vi "GUI.vi"() -> ()   [LabVIEW 2024]
uses:
  <vilib>/Python/Open Anaconda Python Session.vi
panel:
  out "转换完成":bool
  in  "开始转换":bool
  out "运行中":bool
  in  "OCR all pages":bool
  in  "Batch_multiplier":i32(slide) scale=0.0..8.0
  in  "Start page":i32
  in  "Max pages":i32
  in  "PDF directory":path
  out "错误输出":errorcluster
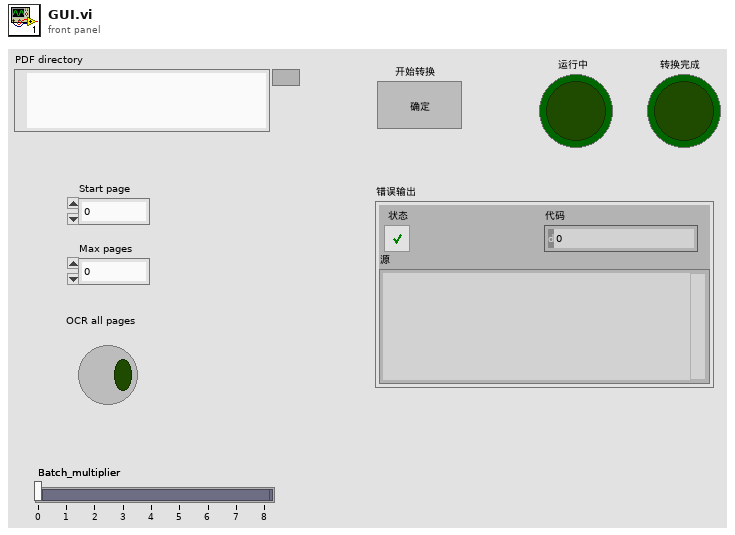
[diagram p1: front panel]
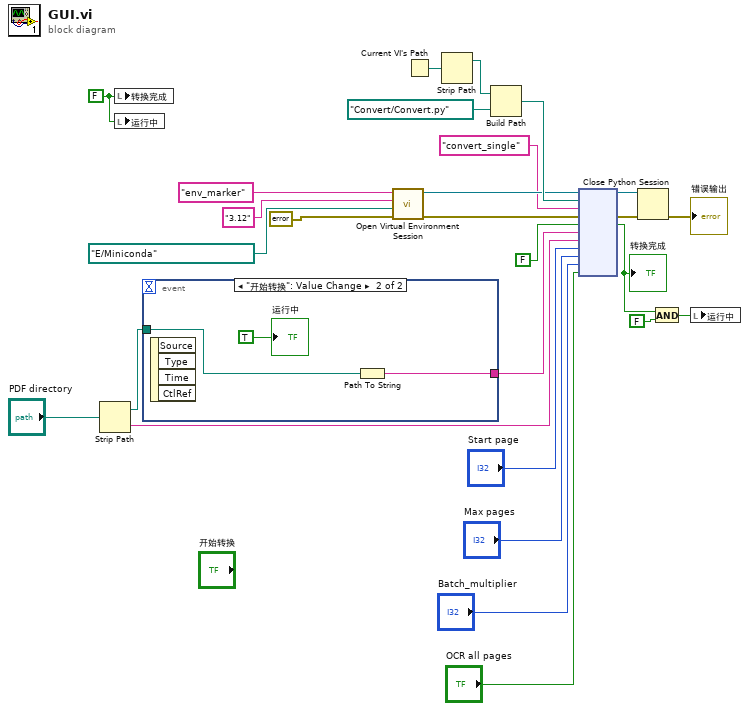
[diagram p0: block diagram]
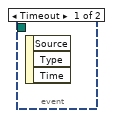
[diagram p2: hidden frame]
diagram:
  w4 = FALSE
  n1 = Strip Path(path="PDF directory") -> (stripped path=w11:path, name=w10:string)
  n2 = local write "转换完成"(w4) -> ()
  n3 = local write "运行中"(w4) -> ()
  n4 = event shown="[1] \"开始转换\": Value Change" {
    selector: _ -> [_ _]
    dyn-events: _ -> [_ _]
    timeout: _ -> [_ _]
    tunnel: [_ w30] -> w16
    tunnel: w11 -> [_ w29]
    event Timeout {
      n5 = event-data() -> ()  [unwired: 1 in, 3 out]
    }
    event "开始转换": Value Change {
      n6 = event-data() -> ()  [unwired: 1 in, 4 out]
      n7 = Path To String(path=w29) -> (string=w30:string)
      "运行中" <- TRUE
    }
  }
  n8 = call-poly <vilib>:"Open Virtual Environment Session.vi"("error in (no error)"=errorcluster {"status"=FALSE, "code"=0, "source"=""} ("错误常量"), "Anaconda path"=path "E:/Miniconda", "Python version"="3.12", "Env name"="env_marker") -> ("error out"=w13:errorcluster, "session out"=w26:refnum<k35>)  [unwired: 6 in]
  n9 = Current VI's Path() -> (path=w15:path)
  n10 = Strip Path(path=w15) -> (stripped path=w14:path)  [unwired: 1 out]
  n11 = Build Path(base path=w14, name or relative path=path "Convert/Convert.py") -> (appended path=w27:path)
  n12 = node(w26, w27, "convert_single", w13, FALSE, w16, w10, "Start page", "Max pages", "Batch_multiplier", "OCR all pages") -> (w19:refnum<k35>, w18:errorcluster, w1:bool)  [unwired: 6 in, 2 out]
  "转换完成" <- w1
  n13 = Close Python Session(session in=w19, error in=w18) -> (11:→"错误输出":errorcluster)
  n14 = And(x=w1, y=FALSE) -> (x .and. y?=w3:bool)
  n15 = local write "运行中"(w3) -> ()
